vi "Purge_Timer.vi"() -> ()   [LabVIEW 2016]
panel:
  in  "stop":bool
  out "Done":bool
  in  "cancel_btn":bool
  out "remaining":dbl
  in  "Purge Time":dbl
  out "Purging":bool
  in  "purge_btn":bool
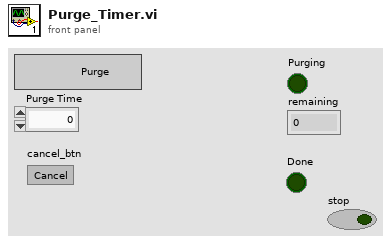
[diagram p1: front panel]
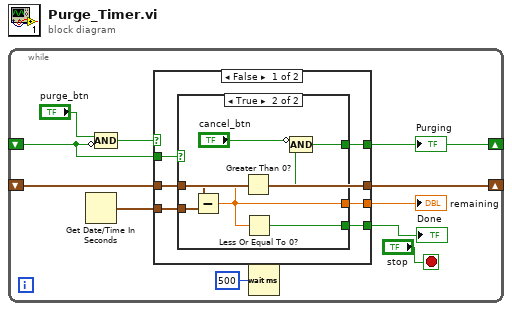
[diagram p0: block diagram]
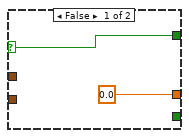
[diagram p2: hidden frame]
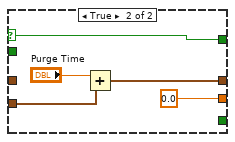
[diagram p3: hidden frame]
diagram:
  n1 = while {
    shift-right: [w10] -> _
    shift-left: _ -> [w8]
    shift-right: [w7] -> _
    shift-left: _ -> [w3]
    stop <- "stop" stop-if-true
    n2 = Get Date/Time In Seconds() -> (seconds since 1Jan1904=w9:timestamp)
    n3 = Compound Arithmetic op=AND("purge_btn", invert w3) -> (w5:bool)
    n4 = case shown="False" w5 {
      selector: w5 -> [_ w30]
      tunnel: [w17 w31] -> w10
      tunnel: w9 -> [w16 w28]
      tunnel: w8 -> [w17 _]
      tunnel: [w13 w30] -> w7
      tunnel: [w15 0.0] -> w4
      tunnel: w3 -> [w14 _]
      tunnel: [w12 _] -> w2
      frame False {
        n5 = case shown="True" w14 {
          selector: w14 -> [w19 _]
          tunnel: w17 -> [_ w26]
          tunnel: w16 -> [_ w25]
          tunnel: [0.0 w21] -> w15
          tunnel: [w19 w22] -> w13
          tunnel: [_ w20] -> w12
          frame False {
          }
          frame True {
            n6 = Subtract(x=w26, y=w25) -> (x-y=w21:dbl)
            n7 = Greater Than 0?(x=w21) -> (x > 0?=w23:bool)
            n8 = Less Or Equal To 0?(x=w21) -> (x <= 0?=w20:bool)
            n9 = Compound Arithmetic op=AND(invert "cancel_btn", w23) -> (w22:bool)
          }
        }
      }
      frame True {
        n10 = Add(x="Purge Time", y=w28) -> (x+y=w31:timestamp)
      }
    }
    "Purging" <- w7
    "remaining" <- w4
    "Done" <- w2
    n11 = Wait (ms)(milliseconds to wait=u32 500) -> ()  [unwired: 1 out]
  }
